vi "Create Knock Command.vi"(8 "error in (no error)":errorcluster, 11 "Section Ptr":T1 format="%.0x") -> (0 "error out":errorcluster, 3 "Parent Ref out":T1 format="%.0x")   [LabVIEW 2016, in "DCM System Explorer.lvlib"]
uses:
  DCM System Explorer.lvlib
  <vilib>/NI Veristand/Custom Device API/Custom Device Item Ref.ctl
  <vilib>/NI Veristand/Custom Device API/Custom Device Channel Type.ctl
  Shared/DCM Constants and GUIDs.vi
  DCM Shared.lvlib
  <vilib>/NI VeriStand/Custom Device API/Custom Device API.lvlib
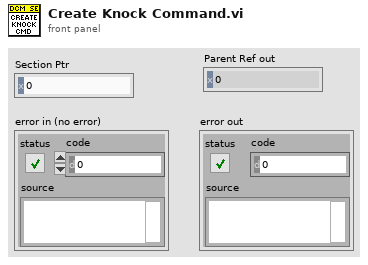
[diagram p1: front panel]
types:
  T1 = typedef "Custom Device API.lvlib/Custom Device Item Ref.ctl" = u64
  T2 = typedef "Custom Device API.lvlib/Custom Device Channel Type.ctl" = enum16{"Input", "Output"}
  T3 = typedef "DCM Shared.lvlib/Channel.ctl" = cluster{"Name":string, "Units":string, "Default":dbl, "Description":string}
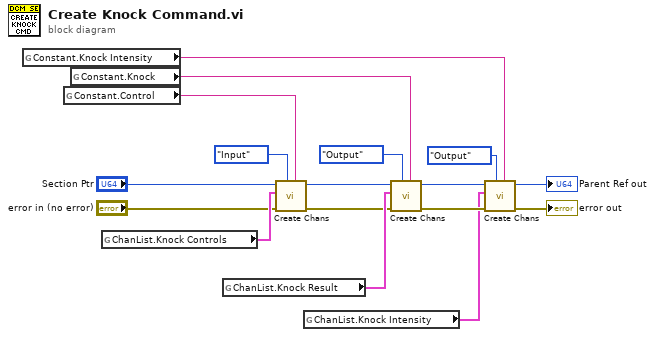
[diagram p0: block diagram]
diagram:
  n1 = global read "DCM Constants and GUIDs.vi" "Constant.Knock Intensity"() -> (w14:string)
  n2 = global read "DCM Constants and GUIDs.vi" "Constant.Control"() -> (w4:string)
  n3 = global read "DCM Constants and GUIDs.vi" "Constant.Knock"() -> (w13:string)
  n4 = global read "DCM Constants and GUIDs.vi" "ChanList.Knock Controls"() -> (w8:T3[])
  n5 = global read "DCM Constants and GUIDs.vi" "ChanList.Knock Result"() -> (w10:T3[])
  n6 = call "Create Chans.vi"("New Section Name (none)"=w4, "Type"=Custom_Device_Channel_Type."Input", "error in (no error)"="error in (no error)", "Channels"=w8, "Section Ptr"="Section Ptr") -> ("error out"=w5:errorcluster, "Section Ptr dup"=w6:T1)  [unwired: 3 in, 2 out]
  n7 = global read "DCM Constants and GUIDs.vi" "ChanList.Knock Intensity"() -> (w9:T3[])
  n8 = call "Create Chans.vi"("New Section Name (none)"=w13, "Type"=Custom_Device_Channel_Type."Output", "error in (no error)"=w5, "Channels"=w10, "Section Ptr"=w6) -> ("error out"=w15:errorcluster, "Section Ptr dup"=w17:T1)  [unwired: 3 in, 2 out]
  n9 = call "Create Chans.vi"("New Section Name (none)"=w14, "Type"=Custom_Device_Channel_Type."Output", "error in (no error)"=w15, "Channels"=w9, "Section Ptr"=w17) -> ("error out"=→"error out":errorcluster, "Section Ptr dup"=→"Parent Ref out":T1)  [unwired: 3 in, 2 out]
